vi "User Code.vi"(8 "error in (no error)":errorcluster, 9 "Image Dst":T1) -> (0 "error out":errorcluster)   [LabVIEW 2019]
uses:
  Simulated Robot/Simulation SubVIs/Simulation SubVIs.lvlib
  <vilib>/vision/NI_Vision_Development_Module.lvlib
  Global 5.vi
  Take_it.vi
  Stage.vi
  Timer.vi
  <vilib>/vision/Image Controls.llb/IMAQ Image.ctl
panel:
  out "relative seconds 2":dbl format="%_19f"
  out "relative seconds":dbl format="%_19f"
  out "Take it!":bool
  out "Stage":i32
  in  "Autopilot":bool
  out "Threshold":T1(plugin-control)
  in  "Value":cluster{i32, i32}(slide)={0, 5} caption="Color Key" scale=0.0..255.0
  in  "Saturation":cluster{i32, i32}(slide)={0, 5} caption="Color Key" scale=0.0..255.0
  in  "Hue":cluster{i32, i32}(slide)={0, 5} caption="Color Key" scale=0.0..255.0
  in  "Backward Button":bool
  in  "Left Button":bool
  in  "Right Button":bool
  in  "Forward Button":bool
  out "right motor ccw velocity (rad/s)":dbl format="%#.3g"
  out "left motor ccw velocity (rad/s)":dbl format="%#.3g"
  in  "Camera Position (rad)":dbl(slide)=-1.0 step=0.01 scale=0.0..-1.5
  out "Raw Image":T1(plugin-control)
  in  "J5 Position (m)":dbl(slide) scale=-0.03..0.01
  in  "J3 Position (m)":dbl(slide)
  in  "J1 Position (m)":dbl(slide) step=0.01
  out "ForwardRight Distance (m)":dbl
  out "ForwardLeft Distance (m)":dbl
  out "Right Distance (m)":dbl
  out "Left Distance (m)":dbl
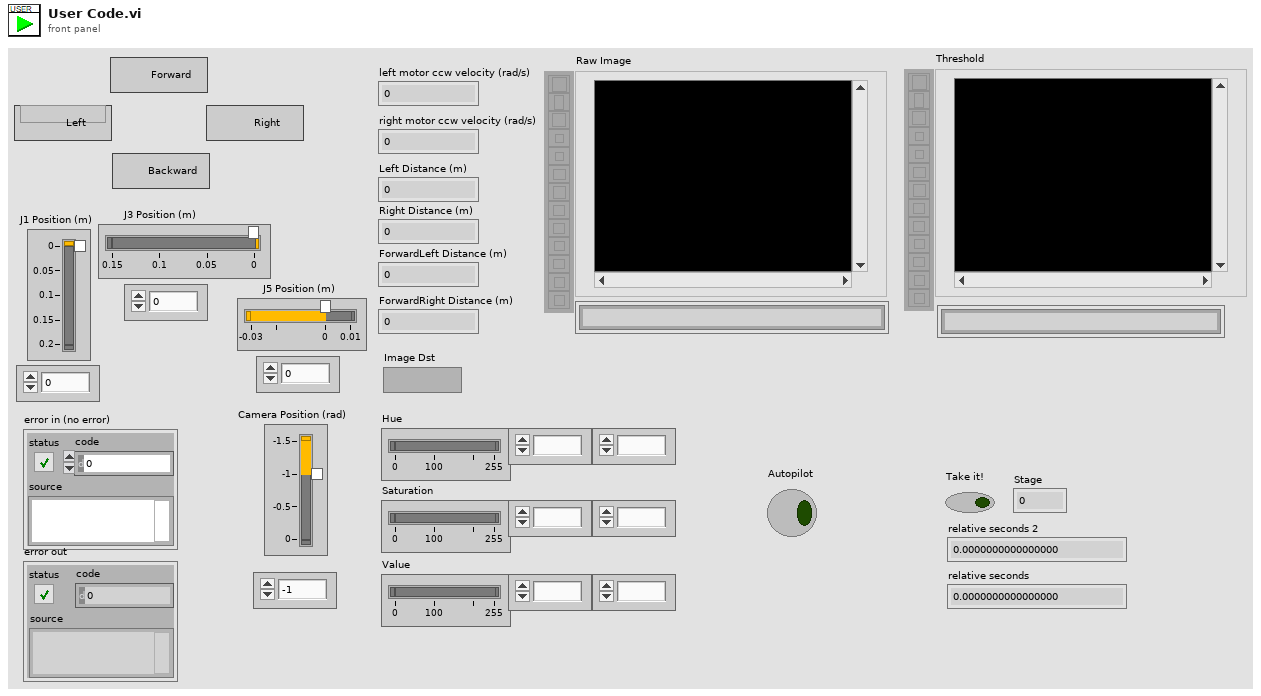
[diagram p1: front panel]
types:
  T1 = typedef "IMAQ Image.ctl" = refnum<image>
  T2 = typedef "Particle Parameters" = i32
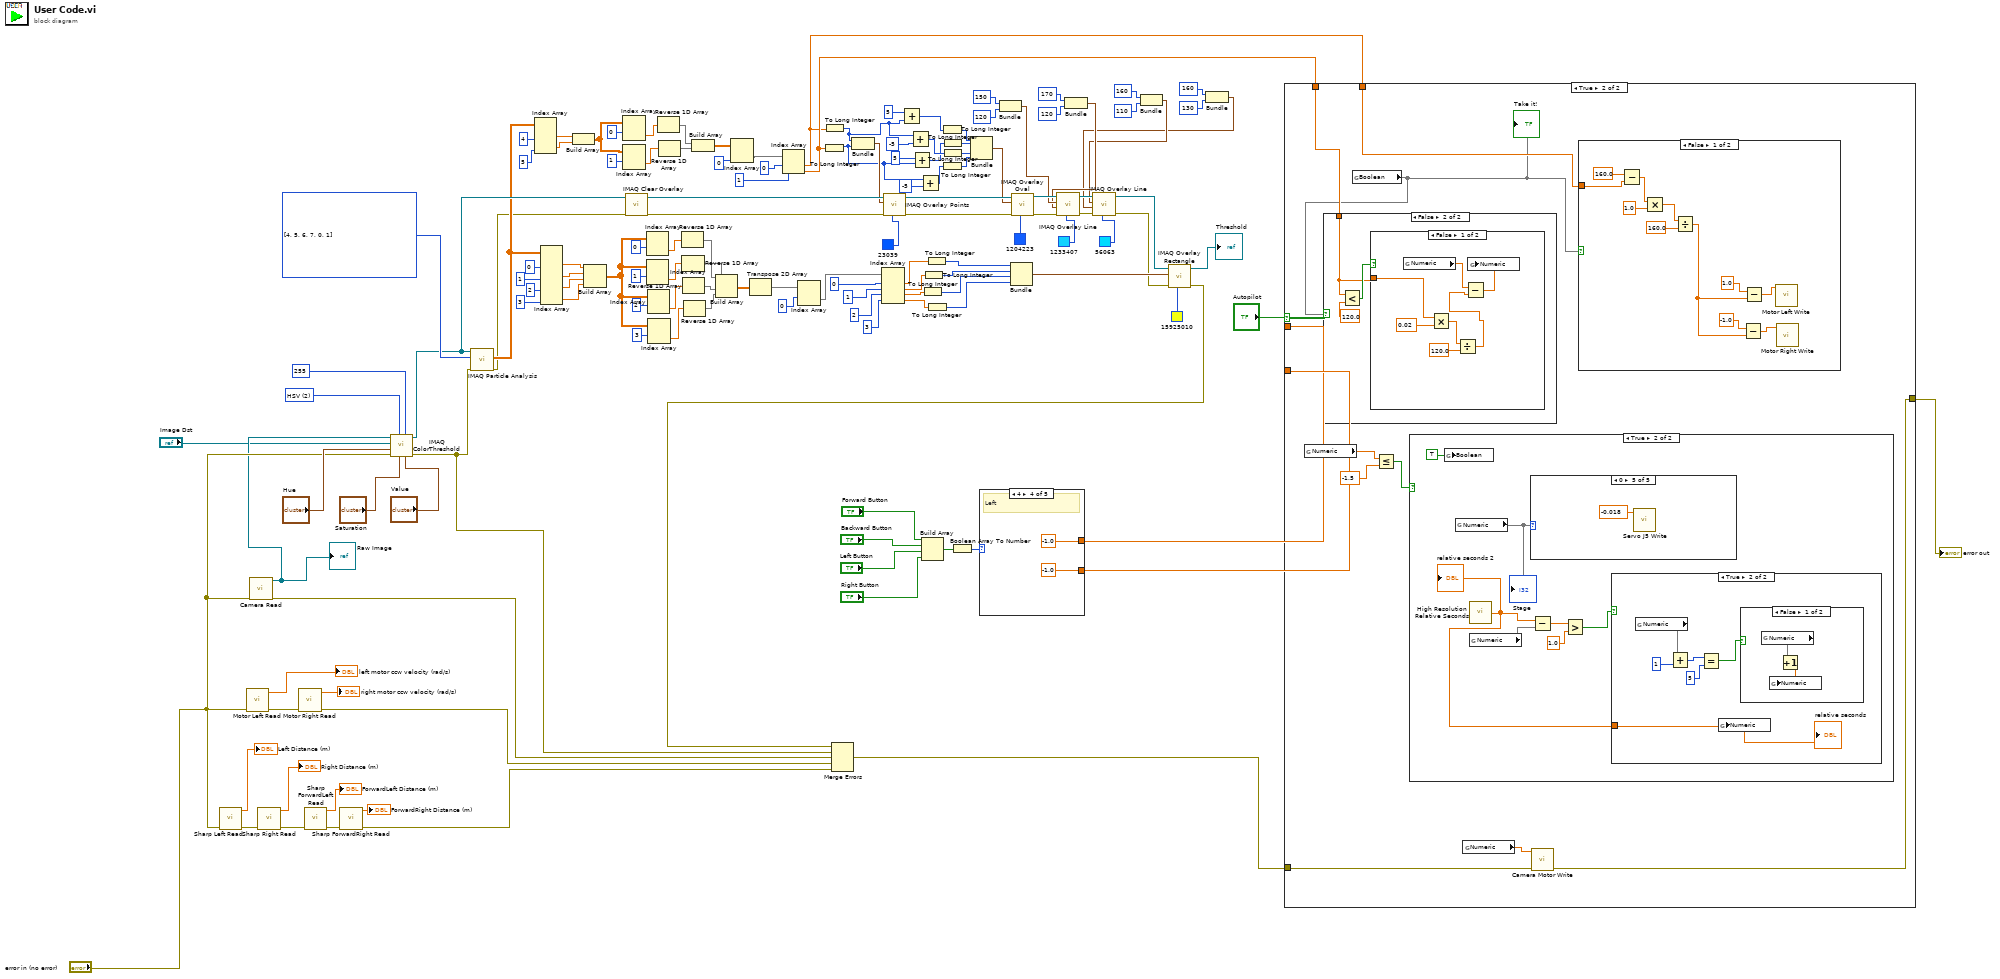
[diagram p0: block diagram]
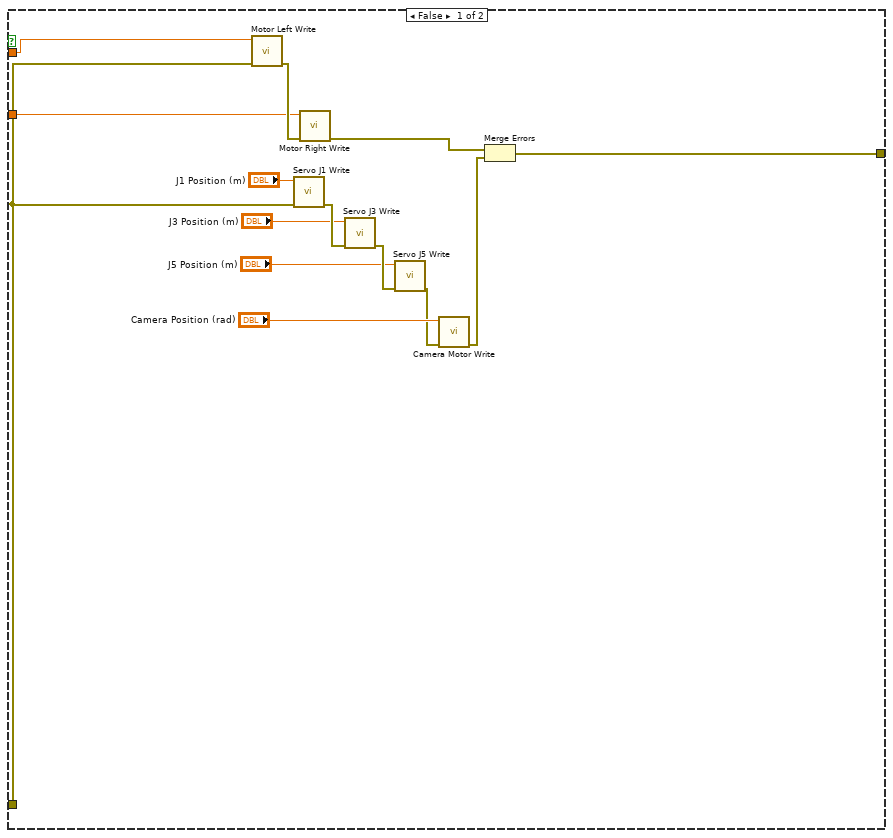
[diagram p2: hidden frame]
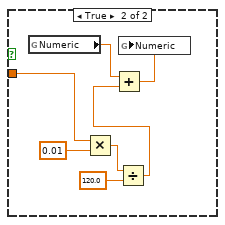
[diagram p4: hidden frame]
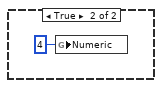
[diagram p7: hidden frame]
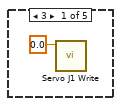
[diagram p8: hidden frame]
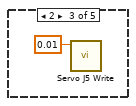
[diagram p10: hidden frame]
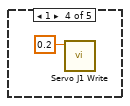
[diagram p11: hidden frame]
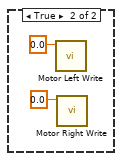
[diagram p12: hidden frame]
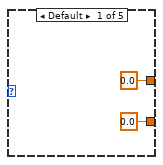
[diagram p13: hidden frame]
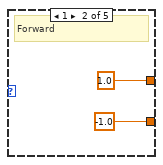
[diagram p14: hidden frame]
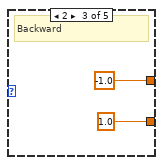
[diagram p15: hidden frame]
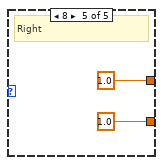
[diagram p16: hidden frame]
diagram:
  w116 = u16 2 items=["RGB", "HSL", "HSV", "HSI"] ("Color Mode")
  w110 = T2[] [4, 5, 6, 7, 0, 1] items=["Center of Mass X", "Center of Mass Y", "First Pixel X", "First Pixel Y", "Bounding Rect Left", "Bounding Rect Top", "Bounding Rect Right", "Bounding Rect Bottom", "Max Feret Diameter Start X", "Max Feret Diameter Start Y", "Max Feret Diameter End X", "Max Feret Diameter End Y", "Max Horiz. Segment Length Left", "Max Horiz. Segment Length Right", "Max Horiz. Segment Length Row", "-", "Bounding Rect Width", "Bounding Rect Height", "Bounding Rect Diagonal", "Perimeter", "Convex Hull Perimeter", "Holes' Perimeter", "Max Feret Diameter", "Equivalent Ellipse Major Axis", "Equivalent Ellipse Minor Axis", "Equivalent Ellipse Minor Axis (Feret)", "Equivalent Rect Long Side", "Equivalent Rect Short Side", "Equivalent Rect Diagonal", "Equivalent Rect Short Side (Feret)", "Average Horiz. Segment Length", "Average Vert. Segment Length", "Hydraulic Radius", "Waddel Disk Diameter", "-", "Area", "Holes' Area", "Particle & Holes' Area", "Convex Hull Area", "Image Area", "-", "Number of Holes", "Number of Horiz. Segments", "Number of Vert. Segments", "-", "Orientation", "Max Feret Diameter Orientation", "-", "% Area/Image Area", "% Area/(Particle & Holes' Area)", "Ratio of Equivalent Ellipse Axes", "Ratio of Equivalent Rect Sides", "-", "Elongation Factor", "Compactness Factor", "Heywood Circularity Factor", "Type Factor", "-", "Sum X", "Sum Y", "Sum XX", "Sum XY", "Sum YY", "Sum XXX", "Sum XXY", "Sum XYY", "Sum YYY", "-", "Moment of Inertia XX", "Moment of Inertia XY", "Moment of Inertia YY", "Moment of Inertia XXX", "Moment of Inertia XXY", "Moment of Inertia XYY", "Moment of Inertia YYY", "Norm. Moment of Inertia XX", "Norm. Moment of Inertia XY", "Norm. Moment of Inertia YY", "Norm. Moment of Inertia XXX", "Norm. Moment of Inertia XXY", "Norm. Moment of Inertia XYY", "Norm. Moment of Inertia YYY", "Hu Moment 1", "Hu Moment 2", "Hu Moment 3", "Hu Moment 4", "Hu Moment 5", "Hu Moment 6", "Hu Moment 7"] ("Pixel Measurements")
  n1 = call "Sharp Left Read.vi"("error in (no error)"="error in (no error)") -> ("error out"=w134:errorcluster, "Left Distance (m)"=→"Left Distance (m)":dbl)  [unwired: 9 in]
  n2 = call "Motor Left Read.vi"("error in (no error)"="error in (no error)") -> ("error out"=w131:errorcluster, "left motor ccw velocity (rad/s)"=→"left motor ccw velocity (rad/s)":dbl)  [unwired: 9 in]
  n3 = call "Camera Read.vi"("error in (no error)"="error in (no error)") -> ("error out"=w126:errorcluster, "Camera Image"=w113:T1)  [unwired: 9 in]
  "Raw Image" <- w113
  n4 = call "Sharp Right Read.vi"("error in (no error)"=w134) -> ("error out"=w133:errorcluster, "Right Distance (m)"=→"Right Distance (m)":dbl)  [unwired: 9 in]
  n5 = call "Motor Right Read.vi"("error in (no error)"=w131) -> ("error out"=w127:errorcluster, "right motor ccw velocity (rad/s)"=→"right motor ccw velocity (rad/s)":dbl)  [unwired: 9 in]
  n6 = call "Sharp ForwardLeft Read.vi"("error in (no error)"=w133) -> ("error out"=w132:errorcluster, "ForwardLeft Distance (m)"=→"ForwardLeft Distance (m)":dbl)  [unwired: 9 in]
  n7 = call "Sharp ForwardRight Read.vi"("error in (no error)"=w132) -> ("error out"=w128:errorcluster, "ForwardRight Distance (m)"=→"ForwardRight Distance (m)":dbl)  [unwired: 9 in]
  n8 = call "IMAQ ColorThreshold"("Blue or Luma or Val or Inten Range"="Value", "Replace Value"=255, "Green or Sat Range"="Saturation", "Color Mode"=w116, "error in (no error)"="error in (no error)", "Red or Hue Range"="Hue", "Image Dst"="Image Dst", "Image Src"=w113) -> ("error out"=w112:errorcluster, "Image Dst Out"=w101:T1)  [unwired: 2 in]
  n9 = call "IMAQ Particle Analysis"("error in (no error)"=w112, "Pixel Measurements"=w110, "Image"=w101) -> ("error out"=w40:errorcluster, "Particle Measurements (Pixels)"=w64:dbl[][])  [unwired: 3 in, 4 out]
  n10 = Index Array(array=w64, index (col) #1=4 ("disabled index (col)"), index (col) #2=5 ("index (col)")) -> (element #1=w56:dbl[], element #2=w55:dbl[])  [unwired: 2 in]
  n11 = Index Array(array=w64, index (col) #1=0 ("disabled index (col)"), index (col) #2=1 ("index (col)"), index (col) #3=2 ("index (col)"), index (col) #4=3 ("index (col)")) -> (element #1=w105:dbl[], element #2=w104:dbl[], element #3=w103:dbl[], element #4=w102:dbl[])  [unwired: 4 in]
  n12 = Build Array(w56, w55) -> (w52:dbl[][])
  n13 = Build Array(w105, w104, w103, w102) -> (w92:dbl[][])
  n14 = Index Array(array=w52, index (row)=0) -> (element=w51:dbl[])  [unwired: 1 in]
  n15 = Index Array(array=w52, index (row)=1) -> (element=w50:dbl[])  [unwired: 1 in]
  n16 = call "IMAQ Clear Overlay"("error in (no error)"=w40, "Image"=w101) -> ("error out"=w39:errorcluster, "Image Out"=w62:T1)  [unwired: 8 in]
  n17 = Index Array(array=w92, index (row)=0) -> (element=w100:dbl[])  [unwired: 1 in]
  n18 = Index Array(array=w92, index (row)=1) -> (element=w99:dbl[])  [unwired: 1 in]
  n19 = Index Array(array=w92, index (row)=2) -> (element=w98:dbl[])  [unwired: 1 in]
  n20 = Index Array(array=w92, index (row)=3) -> (element=w93:dbl[])  [unwired: 1 in]
  n21 = Reverse 1D Array(array=w51) -> (reversed array=w49:dbl[])
  n22 = Reverse 1D Array(array=w50) -> (reversed array=w48:dbl[])
  n23 = Reverse 1D Array(array=w100) -> (reversed array=w96:dbl[])
  n24 = Reverse 1D Array(array=w99) -> (reversed array=w97:dbl[])
  n25 = Reverse 1D Array(array=w98) -> (reversed array=w95:dbl[])
  n26 = Reverse 1D Array(array=w93) -> (reversed array=w94:dbl[])
  n27 = Build Array(w49, w48) -> (w47:dbl[][])
  n28 = Build Array(w96, w97, w95, w94) -> (w87:dbl[][])
  n29 = Index Array(array=w47, index (col)=0 ("index (row)")) -> (element=w61:dbl[])  [unwired: 1 in]
  n30 = Transpose 2D Array(2D array=w87) -> (transposed array=w74:dbl[][])
  n31 = Index Array(array=w61, index #1=0 ("index"), index #2=1 ("index")) -> (element #1=w1:dbl, element #2=w46:dbl)
  n32 = Index Array(array=w74, index (row)=0) -> (element=w73:dbl[])  [unwired: 1 in]
  n33 = To Long Integer(number=w46) -> (32bit integer=w25:i32)
  n34 = To Long Integer(number=w1) -> (32bit integer=w28:i32)
  n35 = Bundle(w28, w25) -> (w57:cluster{i32, i32})  [unwired: 1 in]
  n36 = Index Array(array=w73, index #1=0 ("index"), index #2=1 ("index"), index #3=2 ("index"), index #4=3 ("index")) -> (element #1=w72:dbl, element #2=w71:dbl, element #3=w70:dbl, element #4=w69:dbl)
  n37 = call "IMAQ Overlay Points"("Color"=u32 23039, "error in (no error)"=w39, "Point"=w57, "Image"=w62) -> ("error out"=w38:errorcluster, "Image Out"=w41:T1)  [unwired: 6 in]
  n38 = Add(x=5, y=w28) -> (x+y=w30:i32)
  n39 = Add(x=w28, y=-5) -> (x+y=w29:i32)
  n40 = Add(x=5, y=w25) -> (x+y=w22:i32)
  n41 = Add(x=w25, y=-5) -> (x+y=w23:i32)
  n42 = To Long Integer(number=w70) -> (32bit integer=w78:i32)
  n43 = Build Array("Forward Button", "Backward Button", "Left Button", "Right Button") -> (w125:bool[])
  n44 = To Long Integer(number=w71) -> (32bit integer=w79:i32)
  n45 = To Long Integer(number=w72) -> (32bit integer=w80:i32)
  n46 = To Long Integer(number=w69) -> (32bit integer=w77:i32)
  n47 = To Long Integer(number=w30) -> (32bit integer=w32:i32)
  n48 = To Long Integer(number=w23) -> (32bit integer=w33:i32)
  n49 = To Long Integer(number=w22) -> (32bit integer=w35:i32)
  n50 = To Long Integer(number=w29) -> (32bit integer=w34:i32)
  n51 = Boolean Array To Number(Boolean array=w125) -> (number=w120:u32)
  n52 = Bundle(w32, w35, w34, w33) -> (w36:cluster{i32, i32, i32, i32})  [unwired: 1 in]
  n53 = case shown="4" w120 {
    tunnel: [0.0 ("left motor ccw velocity setpoint (rad/s)") 1.0 ("left motor ccw velocity setpoint (rad/s)") -1.0 ("left motor ccw velocity setpoint (rad/s)") -1.0 ("left motor ccw velocity setpoint (rad/s)") 1.0 ("left motor ccw velocity setpoint (rad/s)")] -> w43
    tunnel: [0.0 ("left motor ccw velocity setpoint (rad/s)") -1.0 ("left motor ccw velocity setpoint (rad/s)") 1.0 ("left motor ccw velocity setpoint (rad/s)") -1.0 ("left motor ccw velocity setpoint (rad/s)") 1.0 ("left motor ccw velocity setpoint (rad/s)")] -> w44
    frame Default {
    }
    frame 1 {
      # "Forward"
    }
    frame 2 {
      # "Backward"
    }
    frame 4 {
      # "Left"
    }
    frame 8 {
      # "Right"
    }
  }
  n54 = Bundle(150, 120) -> (w11:cluster{i32, i32})  [unwired: 1 in]
  n55 = Bundle(w80, w79, w78, w77) -> (w81:cluster{i32, i32, i32, i32})  [unwired: 1 in]
  n56 = call "IMAQ Overlay Oval"("Color"=u32 1204223, "error in (no error)"=w38, "Bounding Rectangle"=w36, "Image"=w41) -> ("error out"=w20:errorcluster, "Image Out"=w21:T1)  [unwired: 6 in]
  n57 = Bundle(170, 120) -> (w8:cluster{i32, i32})  [unwired: 1 in]
  n58 = call "IMAQ Overlay Line"("Color"=u32 1233407, "error in (no error)"=w20, "End Point"=w8, "Start Point"=w11, "Image"=w21) -> ("error out"=w18:errorcluster, "Image Out"=w19:T1)  [unwired: 5 in]
  n59 = Bundle(160, 110) -> (w3:cluster{i32, i32})  [unwired: 1 in]
  n60 = Bundle(160, 130) -> (w2:cluster{i32, i32})  [unwired: 1 in]
  n61 = call "IMAQ Overlay Line"("Color"=u32 56063, "error in (no error)"=w18, "End Point"=w2, "Start Point"=w3, "Image"=w19) -> ("error out"=w17:errorcluster, "Image Out"=w16:T1)  [unwired: 5 in]
  n62 = call "IMAQ Overlay Rectangle"("Color"=u32 15925010, "error in (no error)"=w17, "Rectangle"=w81, "Image"=w16) -> ("error out"=w75:errorcluster, "Image Out"=→"Threshold":T1)  [unwired: 6 in]
  n63 = Merge Errors(w75, w112, w126, w127, w128) -> (w45:errorcluster)
  n64 = case shown="True" "Autopilot" {
    tunnel: w46 -> [_ w168]
    tunnel: w45 -> [w151 w170]
    tunnel: w44 -> [w152 _]
    tunnel: w43 -> [w150 _]
    tunnel: [w149 w169] -> w42
    tunnel: w1 -> [_ w167]
    frame False {
      n65 = call "Motor Left Write.vi"("error in (no error)"=w151, "left motor ccw velocity (rad/s)"=w150) -> ("error out"=w156:errorcluster)  [unwired: 9 in]
      n66 = call "Servo J1 Write.vi"("error in (no error)"=w151, "J1 Position (m)"="J1 Position (m)") -> ("error out"=w157:errorcluster)  [unwired: 9 in]
      n67 = call "Motor Right Write.vi"("error in (no error)"=w156, "right motor ccw velocity (rad/s)"=w152) -> ("error out"=w159:errorcluster)  [unwired: 9 in]
      n68 = call "Servo J3 Write.vi"("error in (no error)"=w157, "J3 Position (m)"="J3 Position (m)") -> ("error out"=w158:errorcluster)  [unwired: 9 in]
      n69 = call "Servo J5 Write.vi"("error in (no error)"=w158, "J5 Position (m)"="J5 Position (m)") -> ("error out"=w160:errorcluster)  [unwired: 9 in]
      n70 = call "Camera Motor Write.vi"("error in (no error)"=w160, "Camera Position (rad)"="Camera Position (rad)") -> ("error out"=w161:errorcluster)  [unwired: 9 in]
      n71 = Merge Errors(w159, w161) -> (w149:errorcluster)
    }
    frame True {
      n72 = global read "Global 5.vi" "Numeric"() -> (w166:dbl)
      n73 = global read "Take_it.vi" "Boolean"() -> (w163)
      "Take it!" <- w163
      n74 = case shown="False" w163 {
        tunnel: w168 -> [_ w172]
        frame True {
        }
        frame False {
          n75 = Less?(x=w172, y=120.0) -> (x < y?=w173:bool)
          n76 = case shown="False" w173 {
            tunnel: w172 -> [w179 w182]
            frame False {
              n77 = global read "Global 5.vi" "Numeric"() -> (w181:dbl)
              n78 = Multiply(x=w179, y=0.02) -> (x*y=w177:dbl)
              n79 = Divide(x=w177, y=120.0) -> (x/y=w175:dbl)
              n80 = Subtract(x=w181, y=w175) -> (x-y=w176:dbl)
              n81 = global write "Global 5.vi" "Numeric"(w176) -> ()
            }
            frame True {
              n82 = global read "Global 5.vi" "Numeric"() -> (w188:dbl)
              n83 = Multiply(x=w182, y=0.01) -> (x*y=w185:dbl)
              n84 = Divide(x=w185, y=120.0) -> (x/y=w183:dbl)
              n85 = Add(x=w188, y=w183) -> (x+y=w184:dbl)
              n86 = global write "Global 5.vi" "Numeric"(w184) -> ()
            }
          }
        }
      }
      n87 = Less Or Equal?(x=w166, y=-1.5) -> (x <= y?=w164:bool)
      n88 = case shown="True" w164 {
        frame False {
        }
        frame True {
          n89 = global write "Take_it.vi" "Boolean"(TRUE ("Boolean")) -> ()
          n90 = global read "Stage.vi" "Numeric"() -> (w194)
          "Stage" <- w194
          n91 = call <vilib>:"High Resolution Relative Seconds.vi"() -> ("relative seconds"=w189:dbl)
          "relative seconds 2" <- w189
          n92 = global read "Timer.vi" "Numeric"() -> (w193)
          n93 = case shown="0" w194 {
            frame 3 {
              n94 = call "Servo J1 Write.vi"("J1 Position (m)"=0.0) -> ()  [unwired: 10 in, 1 out]
            }
            frame Default {
            }
            frame 2 {
              n95 = call "Servo J5 Write.vi"("J5 Position (m)"=0.01) -> ()  [unwired: 10 in, 1 out]
            }
            frame 1 {
              n96 = call "Servo J1 Write.vi"("J1 Position (m)"=0.2) -> ()  [unwired: 10 in, 1 out]
            }
            frame 0 {
              n97 = call "Servo J5 Write.vi"("J5 Position (m)"=-0.018) -> ()  [unwired: 10 in, 1 out]
            }
          }
          n98 = Subtract(x=w189, y=w193) -> (x-y=w192:dbl)
          n99 = Greater?(x=w192, y=1.0) -> (0:w190:bool)
          n100 = case shown="True" w190 {
            tunnel: w189 -> [_ w196]
            frame False {
            }
            frame True {
              n101 = global read "Stage.vi" "Numeric"() -> (w201)
              n102 = Add(x=w201, y=1) -> (x+y=w199:i32)
              n103 = Equal?(x=w199, y=5) -> (x = y?=w198:bool)
              n104 = global write "Timer.vi" "Numeric"(w196) -> ()
              n105 = case shown="False" w198 {
                frame False {
                  n106 = global read "Stage.vi" "Numeric"() -> (w203)
                  n107 = Increment(x=w203) -> (x+1=w202:dbl)
                  n108 = global write "Stage.vi" "Numeric"(w202) -> ()
                }
                frame True {
                  n109 = global write "Stage.vi" "Numeric"(4 ("Numeric")) -> ()
                }
              }
              "relative seconds" <- w196
            }
          }
        }
      }
      n110 = global read "Global 5.vi" "Numeric"() -> (w171:dbl)
      n111 = call "Camera Motor Write.vi"("error in (no error)"=w170, "Camera Position (rad)"=w171) -> ("error out"=w169:errorcluster)  [unwired: 9 in]
      n112 = case shown="False" w163 {
        tunnel: w167 -> [w210 _]
        frame False {
          n113 = Subtract(x=160.0, y=w210) -> (x-y=w209:dbl)
          n114 = Multiply(x=w209, y=1.0) -> (x*y=w218:dbl)
          n115 = Divide(x=w218, y=160.0) -> (x/y=w219:dbl)
          n116 = Subtract(x=-1.0, y=w219) -> (x-y=w217:dbl)
          n117 = Subtract(x=1.0, y=w219) -> (x-y=w216:dbl)
          n118 = call "Motor Left Write.vi"("left motor ccw velocity (rad/s)"=w216) -> ()  [unwired: 10 in, 1 out]
          n119 = call "Motor Right Write.vi"("right motor ccw velocity (rad/s)"=w217) -> ()  [unwired: 10 in, 1 out]
        }
        frame True {
          n120 = call "Motor Left Write.vi"("left motor ccw velocity (rad/s)"=0.0) -> ()  [unwired: 10 in, 1 out]
          n121 = call "Motor Right Write.vi"("right motor ccw velocity (rad/s)"=0.0) -> ()  [unwired: 10 in, 1 out]
        }
      }
    }
  }
  "error out" <- w42
